vi "Core-Init.vi"(8 "error in (no error)":errorcluster, 11 "Engine in":refnum<class "Engine.lvclass">) -> (0 "error out":errorcluster, 3 "Engine out":refnum<class "Engine.lvclass">)   [LabVIEW 2024, in "GLF.lvlib" / "Engine.lvclass"]
uses:
  Engine.lvclass
  Command--cluster.ctl
  Command--enum.ctl
  <vilib>/Saukko/LV SDL3/Sources/SDL3/Init/InitFlags--ring.ctl
  Engine.lvclass/Engine.ctl
  <vilib>/Saukko/LV SDL3/Sources/SDL3/Error/GetError-UiThread.vi
  <vilib>/Utility/error.llb/Error Cluster From Error Code.vi
  <vilib>/Saukko/LV SDL3/Sources/SDL3/Init/Init.lvlib
  <vilib>/Saukko/LV SDL3/Sources/SDL3/Timer/Timer.lvlib
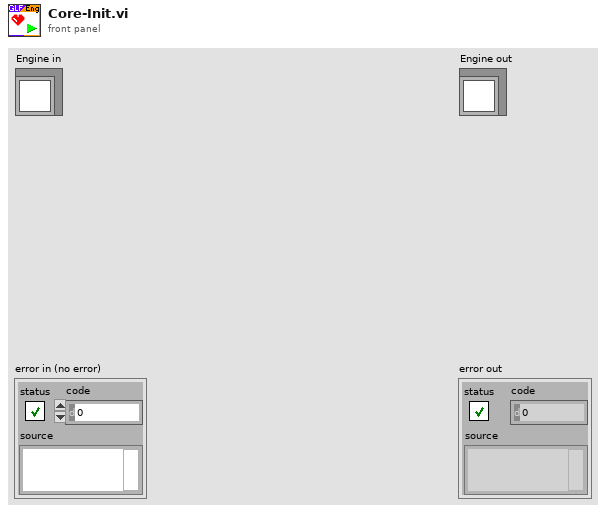
[diagram p1: front panel]
types:
  T1 = typedef "SDL3.lvlib/Init.lvlib/InitFlags--ring.ctl" = u32
  T2 = typedef "GLF.lvlib/Engine.lvclass/Command--cluster.ctl" = cluster{"Cmd":T3, "Data":variant}
  T3 = typedef "GLF.lvlib/Engine.lvclass/Command--enum.ctl" = enum16{"Quit", "Set Data Member"}
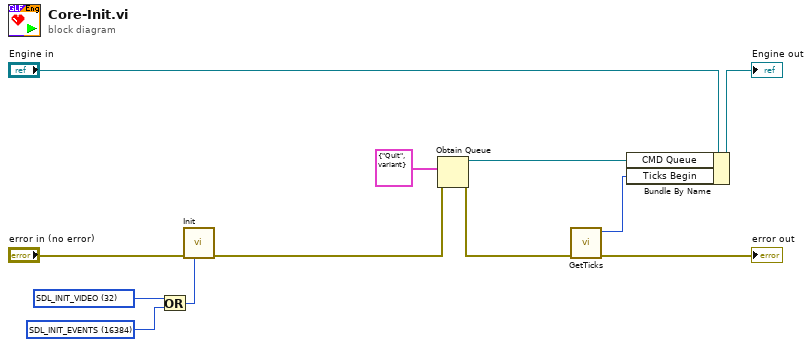
[diagram p0: block diagram]
diagram:
  w4 = T1 16384 items=["NONE"=0, "SDL_INIT_AUDIO"=16, "SDL_INIT_VIDEO"=32, "SDL_INIT_JOYSTICK"=512, "SDL_INIT_HAPTIC"=4096, "SDL_INIT_GAMEPAD"=8192, "SDL_INIT_EVENTS"=16384, "SDL_INIT_SENSOR"=32768, "SDL_INIT_CAMER"=65536] ("y")
  w6 = T1 32 items=["NONE"=0, "SDL_INIT_AUDIO"=16, "SDL_INIT_VIDEO"=32, "SDL_INIT_JOYSTICK"=512, "SDL_INIT_HAPTIC"=4096, "SDL_INIT_GAMEPAD"=8192, "SDL_INIT_EVENTS"=16384, "SDL_INIT_SENSOR"=32768, "SDL_INIT_CAMER"=65536] ("InitFlags")
  n1 = Or(x=w6, y=w4) -> (x .or. y?=w5:T1)
  n2 = call <vilib>:"Init.vi"("InitFlags"=w5, "No Error"="error in (no error)") -> ("error out"=w7:errorcluster)  [unwired: 9 in]
  n3 = Obtain Queue(element data type=T2 {"Cmd"=enum."Quit", "Data"=variant} ("Command"), error in (no error)=w7) -> (queue out=w9:refnum<queue>, error out=w3:errorcluster)  [unwired: 3 in, 1 out]
  n4 = call <vilib>:"GetTicks.vi"("No Error"=w3) -> ("error out"=→"error out":errorcluster, "Ticks [ms]"=w1:u64)  [unwired: 9 in]
  n5 = Bundle By Name(cluster="Engine in", "CMD Queue"=w9, "Ticks Begin"=w1) -> (→"Engine out":refnum<class "Engine.lvclass">)
